vi "Quick Start - Simple - Upload Video.vi"(11 "File Path":path) -> ()   [LabVIEW 2020]
uses:
  Nominal Client/Nominal Client.lvclass
  7453b450-11aa-4de2-86c8-e10972c9b5f7.vi
  faeaf878-661e-4d14-b53d-94c8346d8783.vi
  datasources/target/target.lvclass
  datasources/source/source.lvclass
  datasources/dataset/dataset.lvclass
  nominal types/channelConfig/channelConfig.lvclass
  nominal types/timestampManifest/timestampManifest.lvlib
  3c996d85-85ee-4f1b-8ba4-1d422fd8a5cd.vi
  Nominal Client/upload_ingest.video.vi
  Nominal Client/video.get_ingest_status.vi
  datasources/source/create_s3.vi
  nominal types/timestampManifest/create.noManifest_scale_factor.vi
  Nominal Client/ingest_video.vi
  datasources/target.video/create.new_video.vi
  datasources/target.video/target.video.lvclass
  nominal types/timestampManifest/noManifest/noManifest.lvclass
  C:/code/labview-client/lv_src/nominal types/timestampManifest/timestampManifest/timestampManifest.lvclass
  C:/code/labview-client/lv_src/Nominal Client/datasources/payload/payload.lvclass
  C:/code/labview-client/lv_src/nominal types/timestampManifest/noManifest/noManifest.lvclass
  C:/code/labview-client/lv_src/Nominal Client/datasources/target/target.lvclass
  C:/code/labview-client/lv_src/Nominal Client/datasources/target.video/target.video.lvclass
  datasources/s3/s3.lvclass
  C:/code/labview-client/lv_src/Nominal Client/datasources/source/source.lvclass
  C:/code/labview-client/lv_src/Nominal Client/datasources/s3/s3.lvclass
panel:
  in  "API Token (string or path)":string
  in  "Use Express Function":bool
  in  "Starting time":timestamp format="%<%x %.3X>T"
  out "Progress":dbl(slide) scale=0.0..1.0
  in  "Stop wait":bool
  in  "Wait Until Complete":bool
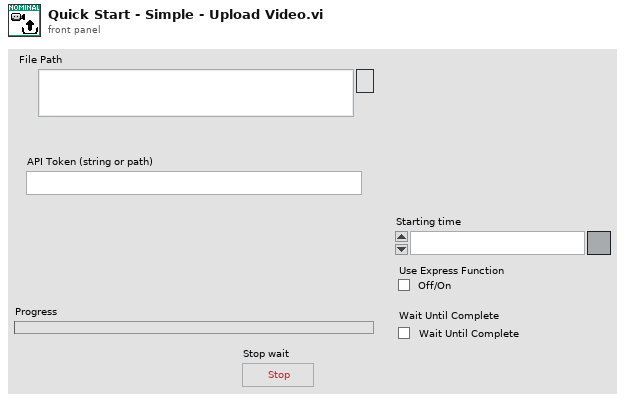
[diagram p1: front panel]
types:
  T1 = cluster{"dataset":refnum<class "dataset.lvclass">, "channelConfig":refnum<class "channelConfig.lvclass">}
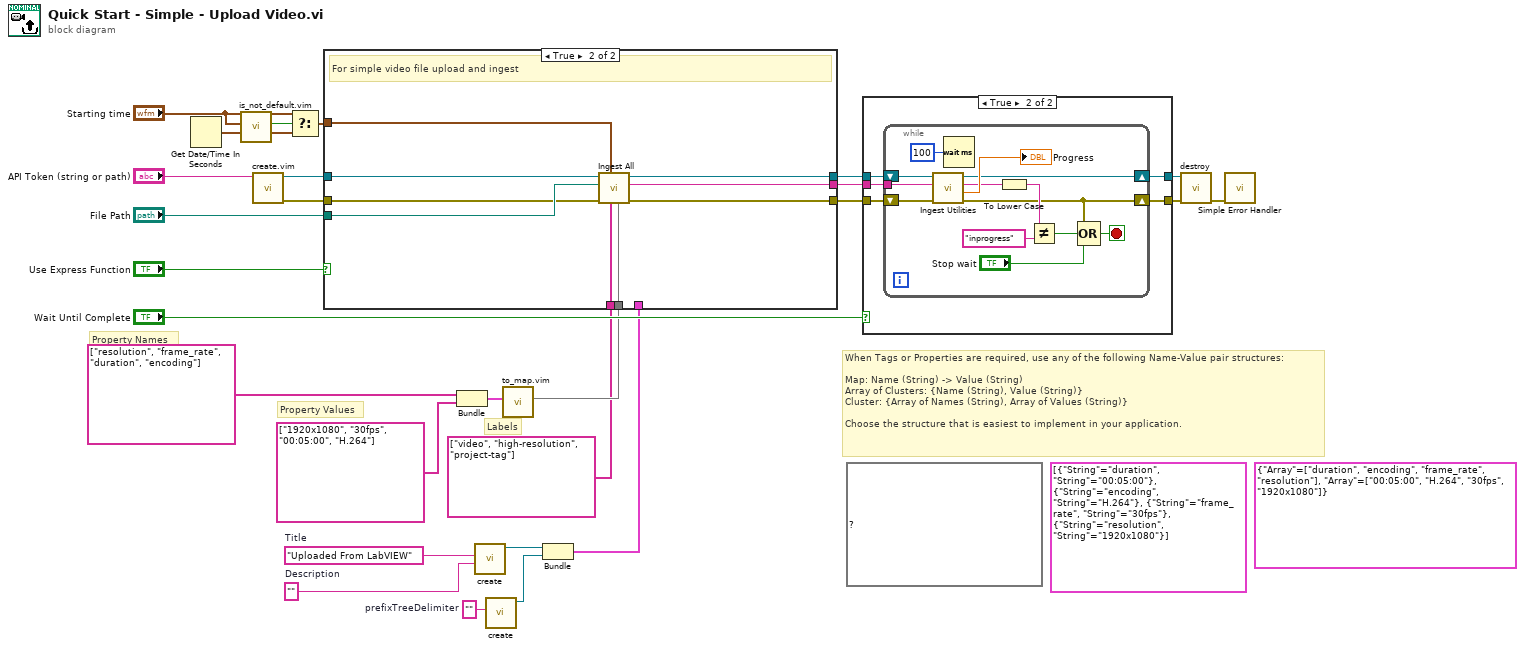
[diagram p0: block diagram]
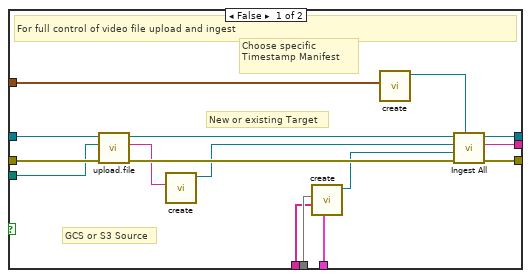
[diagram p2: hidden frame]
diagram:
  w10 = ""  # prefixTreeDelimiter
  w12 = "Uploaded From LabVIEW"  # Title
  w11 = ""  # Description
  (unwired) cluster{"Array":string[], "Array":string[]} {"Array"=["duration", "encoding", "frame_rate", "resolution"], "Array"=["00:05:00", "H.264", "30fps", "1920x1080"]} ("output cluster")
  (unwired) cluster{"String":string, "String":string}[] [{"String"="duration", "String"="00:05:00"}, {"String"="encoding", "String"="H.264"}, {"String"="frame_rate", "String"="30fps"}, {"String"="resolution", "String"="1920x1080"}] ("Array")
  (unwired) map{string, string} {"duration"="00:05:00", "encoding"="H.264", "frame_rate"="30fps", "resolution"="1920x1080"} ("Map out")
  # "When Tags or Properties are required, use any of the following Name-Value pair structures:\n\nMap: Name (String) -> Value (String)\nArray of Clusters: {Name (String), Value (String)}\nCluster: {Array of Names (String), Array of Values (String)}\n\nChoose the structure that is easiest to implement in your application."
  # "Labels"
  # "Property Values"
  # "Property Names"
  n1 = Get Date/Time In Seconds() -> (seconds since 1Jan1904=w3:timestamp)
  n2 = call "is_not_default.vim"("data"="Starting time") -> ("Not Default"=w5:bool)  [unwired: 10 in]
  n3 = call "create.vim"("API Token (string or path)"="API Token (string or path)") -> ("error out"=w26:errorcluster, "Nominal Client"=w27:refnum<class "Nominal Client.lvclass">)  [unwired: 9 in]
  n4 = Select(t="Starting time", s=w5, f=w3) -> (s? t:f=w2:timestamp)
  n5 = Bundle("Labels"=string[] ["resolution", "frame_rate", "duration", "encoding"], "Labels"=string[] ["1920x1080", "30fps", "00:05:00", "H.264"]) -> (w18:cluster{"Labels":string[], "Labels":string[]})  [unwired: 1 in]
  n6 = call "create.vi"("Description"=w11, "Name"=w12) -> ("dataset"=w9:refnum<class "dataset.lvclass">)  [unwired: 9 in]
  n7 = call "create.vi"("prefixTreeDelimiter"=w10) -> ("channelConfig"=w8:refnum<class "channelConfig.lvclass">)  [unwired: 10 in]
  n8 = call "to_map.vim"("Map"=w18) -> ("Map out"=w14:map{string, string})  [unwired: 10 in]
  n9 = Bundle("dataset"=w9, "channelConfig"=w8) -> (w7:T1)  [unwired: 1 in]
  n10 = case shown="True" "Use Express Function" {
    tunnel: w27 -> [w43 w52]
    tunnel: w26 -> [w42 w50]
    tunnel: "File Path" -> [w41 w51]
    tunnel: [w38 w47] -> w17
    tunnel: [w37 w49] -> w16
    tunnel: [w36 w48] -> w15
    tunnel: w14 -> [w32 w45]
    tunnel: string[] ["video", "high-resolution", "project-tag"] ("Labels") -> [w31 w46]
    tunnel: w7 -> [w30 _]
    tunnel: w2 -> [w29 w44]
    frame False {
      # "GCS or S3 Source"
      # "New or existing Target"
      # "Choose specific Timestamp Manifest"
      # "For full control of video file upload and ingest"
      n11 = call "upload.file.vi"("error in"=w42, "File"=w41, "Nominal Client in"=w43) -> ("error out"=w39:errorcluster, "Path to S3 File"=w34:string, "Nominal Client out"=w40:refnum<class "Nominal Client.lvclass">)  [unwired: 6 in]
      n12 = call-poly "create.vi"("Path"=w34) -> ("source"=w33:refnum<class "s3.lvclass">)  [unwired: 10 in]
      n13 = call-poly "create.vi"("Optional"=w30, "Labels"=w31, "Properties"=w32) -> ("target video"=w35:refnum<class "target.video.lvclass">)  [unwired: 7 in, 1 out]
      n14 = call-poly "create.vi"("startingTimestamp"=w29) -> ("Timestamp Manifest"=w28:refnum<class "noManifest.lvclass">)  [unwired: 10 in]
      n15 = call-poly "Ingest All.vi"("Timestamp Manifest"=w28, "error in"=w39, "Target"=w35, "Source"=w33, "Nominal Client in"=w40) -> ("error out"=w37:errorcluster, "videoRid"=w36:string, "Nominal Client out"=w38:refnum<class "Nominal Client.lvclass">)  [unwired: 3 in, 1 out]
    }
    frame True {
      # "For simple video file upload and ingest"
      n16 = call-poly "Ingest All.vi"("Properties"=w45, "Labels"=w46, "Time Stamp"=w44, "error in"=w50, "File Path"=w51, "Nominal Client in"=w52) -> ("error out"=w49:errorcluster, "videoRid"=w48:string, "Nominal Client out"=w47:refnum<class "Nominal Client.lvclass">)  [unwired: 3 in]
    }
  }
  n17 = case shown="True" "Wait Until Complete" {
    tunnel: w17 -> [w53 w59]
    tunnel: w16 -> [w54 w58]
    tunnel: [w54 w57] -> w25
    tunnel: [w53 w56] -> w24
    tunnel: w15 -> [_ w55]
    frame False {
    }
    frame True {
      n18 = while {
        shift-right: [w60] -> w56
        shift-left: w59 -> [w66]
        shift-right: [w63] -> w57
        shift-left: w58 -> [w64]
        tunnel: w55 -> [w65]
        stop <- w68 stop-if-true
        n19 = call-poly "Ingest Utilities.vi"("error in"=w64, "Video RID"=w65, "Nominal Client in"=w66) -> ("error out"=w63:errorcluster, "Progress (0-1)"=→"Progress":dbl, "Status"=w61:string, "Nominal Client out"=w60:refnum<class "Nominal Client.lvclass">)  [unwired: 5 in]
        n20 = Wait (ms)(milliseconds to wait=u32 100) -> ()  [unwired: 1 out]
        n21 = To Lower Case(string=w61) -> (all lower case string=w71:string)
        n22 = Not Equal?(x=w71, y="inprogress") -> (x != y?=w70:bool)
        n23 = Compound Arithmetic op=OR(w63, w70, "Stop wait") -> (w68:bool)
      }
    }
  }
  n24 = call "destroy.vi"("error in"=w25, "Nominal Client"=w24) -> ("error out"=w21:errorcluster)  [unwired: 9 in]
  n25 = call <vilib>:"Simple Error Handler.vi"("error in (no error)"=w21) -> ()  [unwired: 4 in, 5 out]
